vi "HT.vi"(1 "Ctl Refnum 2":refnum<vi>, 2 "Ctl Refnum":refnum<vi>, 3 "Function (0: Cp-D)":u16(ring) items=["Cp-D", "Cp-Q", "Cp-G", "Cp-Rp", "Cs-D", "Cs-Q", "Cs-Rs", "Lp-D", "Lp-Q", "Lp-G", "Lp-Rp", "Lp-Rdc", "Ls-D", "Ls-Q", "Ls-Rs", "Ls-Rdc", "R-X", "Z-thd", "Z-thr", "G-B", "Y-thd", "Y-thr", "Vdc-Idc"], 8 "error in (no error)":errorcluster caption="错误输入（无错误）", 9 "Cluster":T2, 10 "Cluster 2":T1={"开始温度H"=26.0, "变温速率H"=5.0, "结束温度H"=150.0, "簇"={"测试频率"=1000.0, "测试频率 2"=1000.0, "测试频率 3"=1000.0, "测试频率 4"=1000.0}}, 11 "Cluster 3":cluster{"文件路径H：  ":path, "表格数据路径： ":path}={"文件路径H：  "=path "C:/Users/shipeng/Desktop/HTCT TEST", "表格数据路径： "=path "C:/Users/shipeng/Desktop/LT Dielectric measurement"}) -> (0 "错误输出":cluster{"状态":bool, "代码":i32, "源":string})   [LabVIEW 2017]
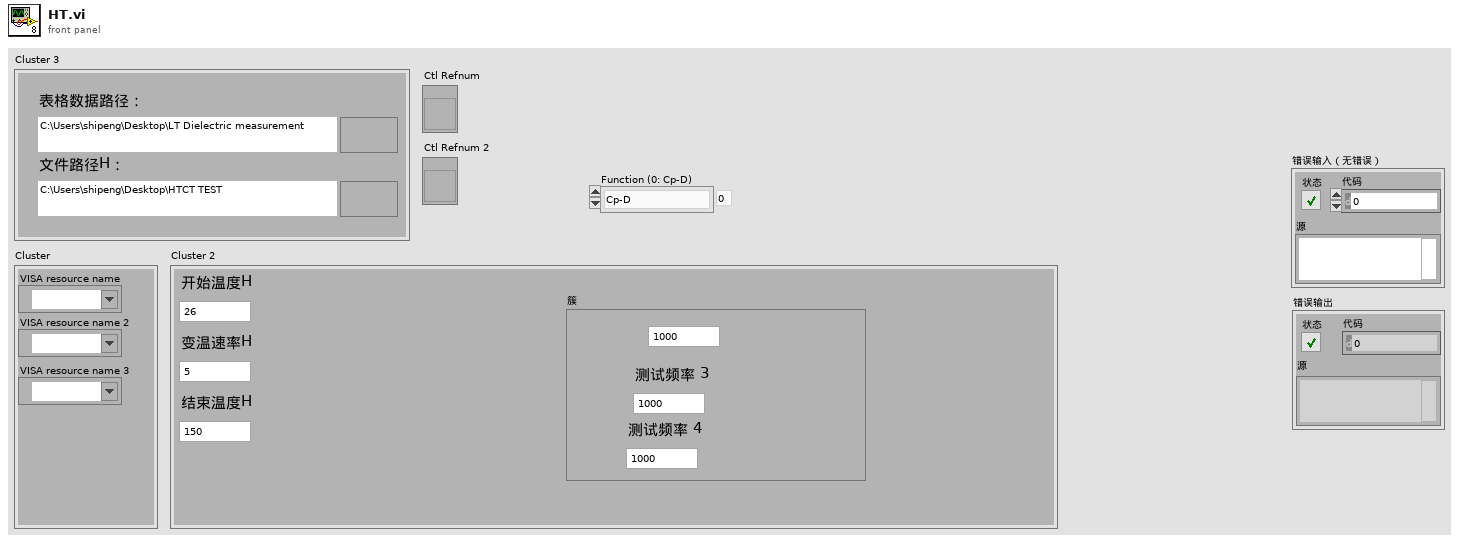
[diagram p1: front panel]
types:
  T1 = cluster{"开始温度H":dbl, "变温速率H":dbl, "结束温度H":dbl, "簇":cluster{"测试频率":dbl, "测试频率 2":dbl, "测试频率 3":dbl, "测试频率 4":dbl}}
  T2 = cluster{"VISA resource name":refnum<visa-resource-name>, "VISA resource name 2":refnum<visa-resource-name>, "VISA resource name 3":refnum<visa-resource-name>}
  T3 = enum16{"open", "replace", "create", "open or create", "replace or create", "replace or create with confirmation"}
  T4 = cluster{"测试频率":dbl, "测试频率 2":dbl, "测试频率 3":dbl, "测试频率 4":dbl}
  T5 = cluster{"结束温度H":dbl, "变温速率H":dbl, "簇":cluster{"测试频率":dbl, "测试频率 2":dbl, "测试频率 3":dbl, "测试频率 4":dbl}}
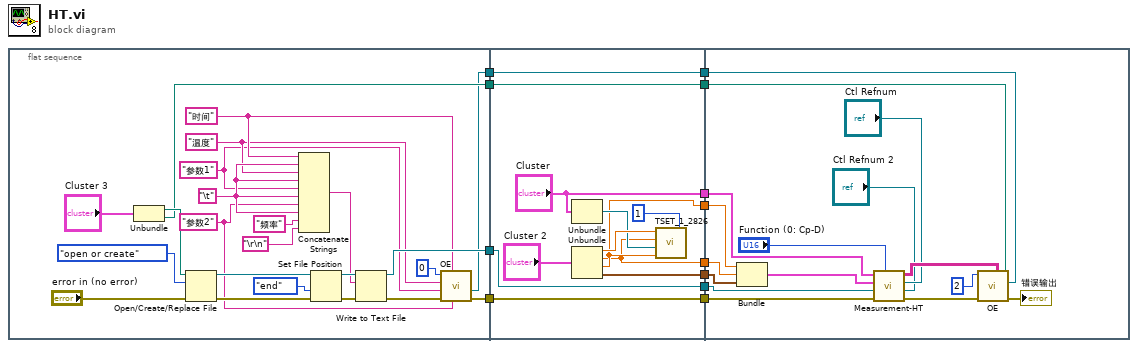
[diagram p0: block diagram]
diagram:
  n1 = flat-sequence {
    tunnel: [w13] -> w8
    tunnel: [w26] -> w7
    tunnel: [w14] -> w6
    tunnel: [w21] -> w5
    tunnel: w7 -> [w46]
    tunnel: [w46] -> w12
    tunnel: [w45] -> w11
    tunnel: w8 -> [w45]
    tunnel: w6 -> [w44]
    tunnel: [w44] -> w10
    tunnel: [w43] -> w9
    tunnel: w5 -> [w43]
    tunnel: [w39] -> w4
    tunnel: [w38] -> w3
    tunnel: [w37] -> w2
    tunnel: ["Cluster"] -> w1
    tunnel: w12 -> [w62]
    tunnel: w11 -> [w63]
    tunnel: w10 -> [w60]
    tunnel: w9 -> [w59]
    tunnel: w4 -> [w52]
    tunnel: w3 -> [w51]
    tunnel: w2 -> [w50]
    tunnel: w1 -> [w49]
    frame #0 {
      w17 = "参数2" ("字符串")
      w18 = "参数1" ("字符串")
      w19 = "温度" ("字符串")
      w29 = "\t"
      w20 = "时间" ("字符串")
      n2 = Unbundle("Cluster 3") -> ("文件路径H："=w22:path, "表格数据路径："=w21:path)
      n3 = Open/Create/Replace File(file path (use dialog)=w22, error in="error in (no error)", operation (0:open)=T3."open or create" ("操作(0:open)")) -> (refnum out=w33:refnum<file>, error out=w32:errorcluster)  [unwired: 1 in, 3 out]
      n4 = Concatenate Strings(w20, w29, w19, w29, w18, w29, w17, w29, "频率" ("字符串"), "\r\n") -> (w31:string)
      n5 = Set File Position(refnum=w33, from (0:start)=enum16{"start", "end", "current"}."end" ("自（0:起始）"), error in=w32) -> (refnum out=w34:refnum<file>, error out=w35:errorcluster)  [unwired: 1 out]
      n6 = Write to Text File(file (use dialog)=w34, text=w31, error in=w35) -> (refnum out=w26:refnum<file>, error out=w15:errorcluster)  [unwired: 2 out]
      n7 = call "OE.vi"("String 4"=w17, "String"=w20, "error in (no error)"=w15, "String 3"=w18, "String 2"=w19, "Numeric"=0) -> ("error out"=w13:errorcluster, "report out"=w14:refnum<class "NI_report.lvclass">)  [unwired: 3 in, 1 out]
    }
    frame #1 {
      n8 = Unbundle("Cluster") -> ("VISA resource name 2"=w40:refnum<visa-resource-name>)  [unwired: 2 out]
      n9 = Unbundle("Cluster 2") -> ("开始温度H"=w42:dbl, "变温速率H"=w38:dbl, "结束温度H"=w39:dbl, "簇"=w37:T4)
      n10 = call "TSET_1_2826.vi"("Address No."=i8 1, "T-Ending, C"=w39, "VISA resource name"=w40, "cooling/heating rate, C/min"=w38, "T-Starting, C"=w42) -> ()
    }
    frame #2 {
      n11 = Bundle("结束温度H"=w52, "变温速率H"=w51, "簇"=w50) -> (w61:T5)  [unwired: 1 in]
      n12 = call "Measurement-HT.vi"("Ctl Refnum 2"="Ctl Refnum 2", "Ctl Refnum"="Ctl Refnum", "Function (0: Cp-D)"="Function (0: Cp-D)", "error in (no error)"=w63, "Byte Stream File Refnum"=w62, "Cluster 2"=w61, "Cluster"=w49) -> ("error out"=w57:errorcluster, "Array"=w58:string[][])  [unwired: 3 in]
      n13 = call "OE.vi"("report in"=w60, "表格数据路径："=w59, "Array"=w58, "error in (no error)"=w57, "Numeric"=i8 2 ("Address No.")) -> ("error out"=→"错误输出":errorcluster)  [unwired: 4 in, 2 out]
    }
  }
